vi "Get Session Management Service Address.vi"(8 "error in (no error)":errorcluster) -> (0 "error out":errorcluster, 3 "address":string)   [LabVIEW 2020]
uses:
  Discovery Client_lv/MeasurementLink Discovery Client/RPC Messages/ni_measurementlink_discovery_v1_ResolveServiceRequest.ctl
  Discovery Client_lv/MeasurementLink Discovery Client/MeasurementLink Discovery Client.lvlib
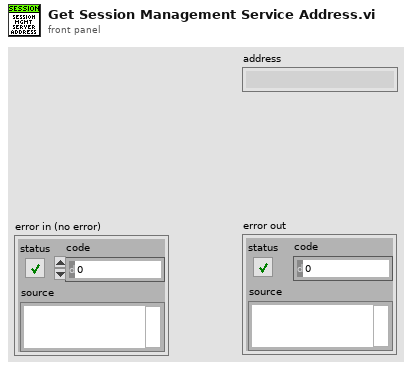
[diagram p1: front panel]
types:
  T1 = typedef "MeasurementLink Discovery Client.lvlib/ni_measurementlink_discovery_v1_ResolveServiceRequest.ctl" = cluster{"provided_interface":string, "service_class":string}
  T2 = typedef "MeasurementLink Discovery Client.lvlib/ni_measurementlink_discovery_v1_ServiceLocation.ctl" = cluster{"location":string, "insecure_port":string, "ssl_authenticated_port":string}
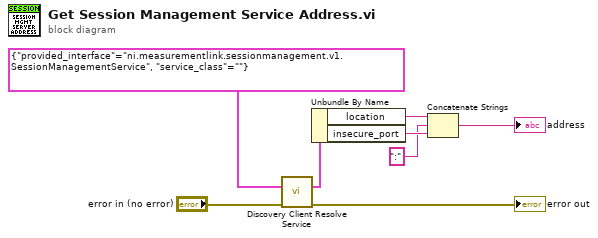
[diagram p0: block diagram]
diagram:
  n1 = call "Discovery Client Resolve Service.vi"("Request Data"=T1 {"provided_interface"="ni.measurementlink.sessionmanagement.v1.SessionManagementService", "service_class"=""}, "error in (no error)"="error in (no error)") -> ("Response Data"=w6:T2, "error out"=→"error out":errorcluster)  [unwired: 12 in]
  n2 = Unbundle By Name(w6) -> ("location"=w5:string, "insecure_port"=w4:string)
  n3 = Concatenate Strings(w5, ":" ("string"), w4) -> (→"address":string)
